vi "GetReference.vi"(8 "error in (no error)":errorcluster, 11 "Footnote in":refnum<class "FootnoteReference.lvclass">) -> (0 "error out":errorcluster, 2 "Reference":string, 3 "Footnote out":refnum<class "FootnoteReference.lvclass">)   [LabVIEW 2021, in "LvMarkdown.lvlib" / "FootnoteReference.lvclass"]
uses:
  FootnoteReference.lvclass
  FootnoteReference.lvclass/FootnoteReference.ctl
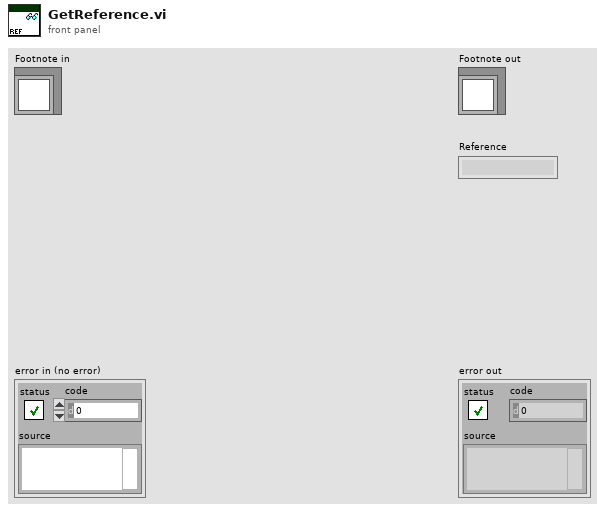
[diagram p1: front panel]
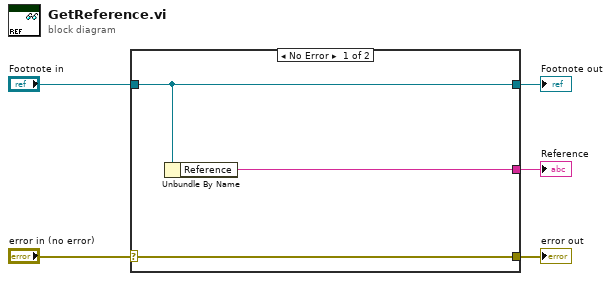
[diagram p0: block diagram]
diagram:
  n1 = case shown="No Error" "error in (no error)" {
    selector: "error in (no error)" -> [w8 w9]
    tunnel: [w8 w9] -> w4
    tunnel: [w7 w10] -> w2
    tunnel: "Footnote in" -> [w7 w10]
    tunnel: [w6 _] -> w1
    frame No Error {
      n2 = Unbundle By Name(w7) -> ("Reference"=w6:string)
    }
    frame Error {
    }
  }
  "error out" <- w4
  "Footnote out" <- w2
  "Reference" <- w1
